vi "check if done HC.vi"(8 "error in (no error)":errorcluster, 11 "Autofocus in":refnum<class "Autofocus.lvclass">) -> (0 "error out":errorcluster, 3 "Autofocus out":refnum<class "Autofocus.lvclass">)   [LabVIEW 2012, in "Autofocus.lvclass"]
uses:
  Autofocus.lvclass
  Autofocus.lvclass/Autofocus.ctl
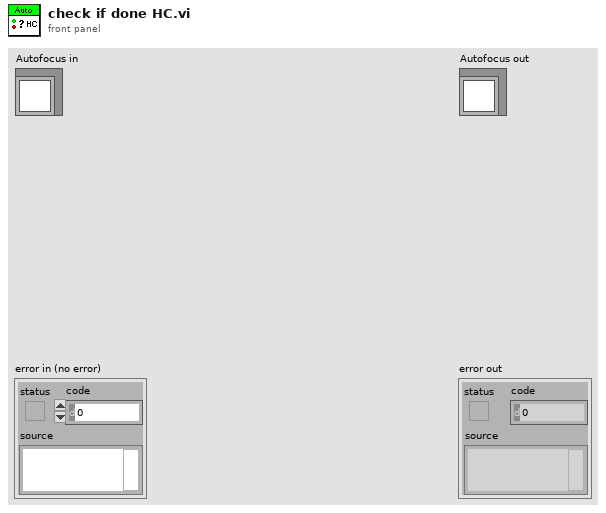
[diagram p1: front panel]
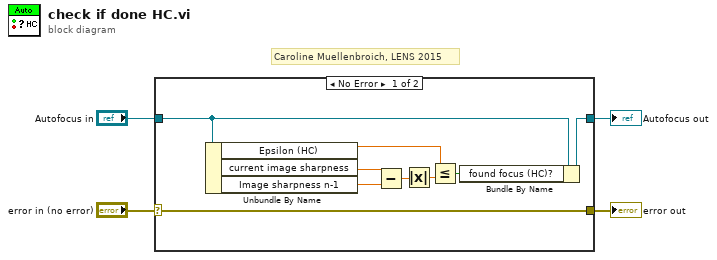
[diagram p0: block diagram]
diagram:
  # "Caroline Muellenbroich, LENS 2015"
  n1 = case shown="No Error" "error in (no error)" {
    selector: "error in (no error)" -> [w13 w15]
    tunnel: [w13 w15] -> w3
    tunnel: [w7 w14] -> w1
    tunnel: "Autofocus in" -> [w9 w14]
    frame No Error {
      n2 = Unbundle By Name(w9) -> ("Epsilon (HC)"=w10:dbl, "current image sharpness"=w12:dbl, "Image sharpness n-1"=w11:dbl)
      n3 = Subtract(x=w12, y=w11) -> (x-y=w6:dbl)
      n4 = Absolute Value(x=w6) -> (abs(x)=w5:dbl)
      n5 = Less Or Equal?(x=w10, y=w5) -> (x <= y?=w8:bool)
      n6 = Bundle By Name(cluster=w9, "found focus (HC)?"=w8) -> (w7:refnum<class "Autofocus.lvclass">)
    }
    frame Error {
    }
  }
  "error out" <- w3
  "Autofocus out" <- w1
